vi "emi_Loop Timing & monitor.vi"() -> (8 "Number of calls":u32, 10 "Time Since Previous call":u32)   [LabVIEW 2010]
doc: "Place in loop to see time per iteration, and numbr of iterations. Reentrent and subroutin priority"
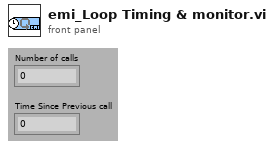
[diagram p1: front panel]
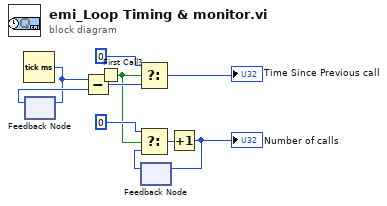
[diagram p0: block diagram]
diagram:
  n1 = Tick Count (ms)() -> (millisecond timer value=w8:u32)
  n2 = feedback-in #1(w8) -> ()
  n3 = feedback #1() -> (w9:u32)  [unwired: 1 out]
  n4 = Subtract(x=w8, y=w9) -> (x-y=w10:u32)
  n5 = First Call?() -> (First Call?: T/F=w1:bool)
  n6 = Select(t=u32 0, s=w1, f=w10) -> (s? t:f=→"Time Since Previous call":u32)
  n7 = feedback #2() -> (w3:u32)  [unwired: 1 out]
  n8 = Select(t=u32 0, s=w1, f=w3) -> (s? t:f=w4:u32)
  n9 = Increment(x=w4) -> (x+1=w2:u32)
  "Number of calls" <- w2
  n10 = feedback-in #2(w2) -> ()
